vi "from-string.vi"(8 "error in (no error)":errorcluster, 10 "uuid-string":string) -> (0 "error out":errorcluster, 3 "UUID out":refnum<class "UUID.lvclass">)   [LabVIEW 2020, in "graph.lvlib" / "UUID.lvclass"]
uses:
  UUID.lvclass
  UUID.lvclass/UUID.ctl
  <vilib>/regexp/Match Regular Expression.xnode
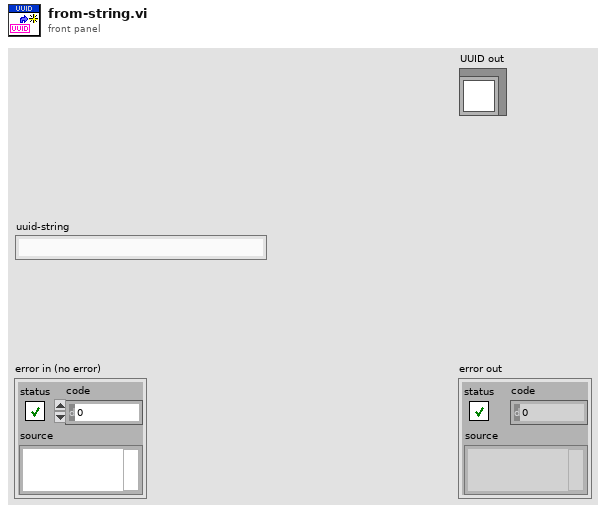
[diagram p1: front panel]
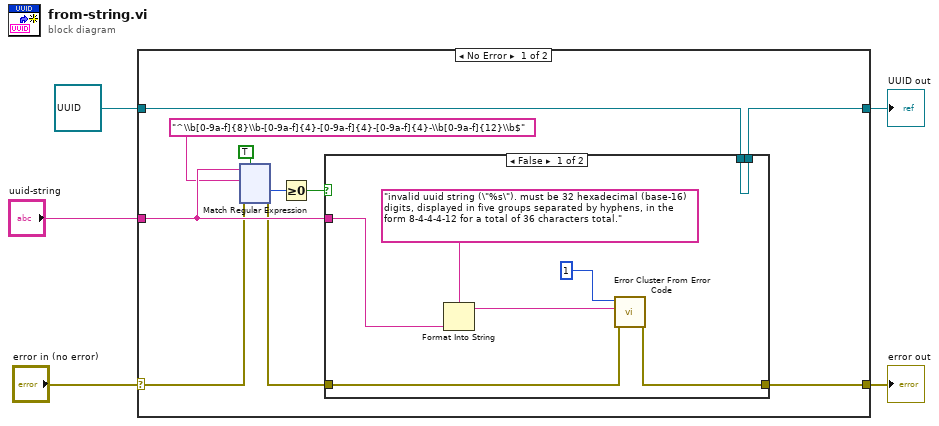
[diagram p0: block diagram]
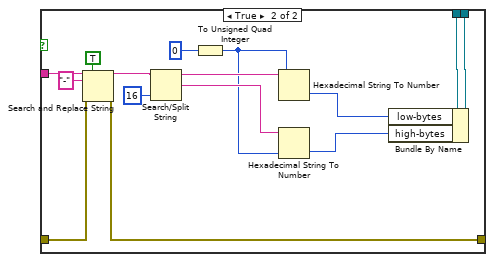
[diagram p2: hidden frame]
diagram:
  n1 = case shown="No Error" "error in (no error)" {
    selector: "error in (no error)" -> [w10 w153]
    tunnel: [w15 w153] -> w4
    tunnel: [w13 w152] -> w2
    tunnel: refnum<class "UUID.lvclass"> refnum ("UUID in") -> [w14 w152]
    tunnel: "uuid-string" -> [w12 _]
    frame No Error {
      n2 = xnode "Match Regular Expression"("input string"=w12, "regular expression"="^\\b[0-9a-f]{8}\\b-[0-9a-f]{4}-[0-9a-f]{4}-[0-9a-f]{4}-\\b[0-9a-f]{12}\\b$", "error in"=w10, "ignore case? (F)"=TRUE) -> ("offset past match"=w7:i32, "error out"=w9:errorcluster)  [unwired: 2 in, 3 out]
      n3 = Greater Or Equal To 0?(x=w7) -> (x >= 0?=w6:bool)
      n4 = case shown="False" w6 {
        tunnel: [w19 w27] -> w15
        tunnel: w14 -> [w22 w26]
        tunnel: [w22 w25] -> w13
        tunnel: w12 -> [w18 w24]
        tunnel: w9 -> [w20 w23]
        frame False {
          n5 = Format Into String(format string="invalid uuid string (\"%s\"). must be 32 hexadecimal (base-16) digits, displayed in five groups separated by hyphens, in the form 8-4-4-4-12 for a total of 36 characters total." ("error message (\"\")"), w18) -> (resulting string=w17:string)  [unwired: 2 in, 1 out]
          n6 = call <vilib>:"Error Cluster From Error Code.vi"("error in (no error)"=w20, "error message (\"\")"=w17, "error code (0)"=1) -> ("error out"=w19:errorcluster)  [unwired: 6 in]
        }
        frame True {
          n7 = Search and Replace String(replace all?=TRUE ("replace all? (F)"), input string=w24, search string="-", error in=w23) -> (result string=w31:string, error out=w27:errorcluster)  [unwired: 4 in, 2 out]
          n8 = Search/Split String(string=w31, offset (0)=16) -> (substring before match=w33:string, match + rest of string=w32:string)  [unwired: 1 in, 1 out]
          n9 = To Unsigned Quad Integer(1:u64 0 ("default (0 U32)")) -> (0:w29:u64)
          n10 = Hexadecimal String To Number(string=w33, default (0uL)=w29) -> (number=w30:u64)  [unwired: 1 in, 1 out]
          n11 = Hexadecimal String To Number(string=w32, default (0uL)=w29) -> (number=w28:u64)  [unwired: 1 in, 1 out]
          n12 = Bundle By Name(cluster=w26, "low-bytes"=w30, "high-bytes"=w28) -> (w25:refnum<class "UUID.lvclass">)
        }
      }
    }
    frame Error {
    }
  }
  "error out" <- w4
  "UUID out" <- w2
